vi "Send Get Temperature WAV.vi"(7 "Message Priority (Normal)":T1=enum."Normal", 8 "error in":errorcluster, 10 "Source":string, 11 "Message Enqueuer":refnum<class "Message Enqueuer.lvclass">) -> (0 "error out":errorcluster, 1 "timed out?":bool, 2 "Reply":variant, 3 "Message Enqueuer out":refnum<class "Message Enqueuer.lvclass">)   [LabVIEW 2024, in "Thermometer Multichannel Worker.lvlib" / "Get Temperature WAV Msg.lvclass"]
doc: "This VI sends the message to an actor."
uses:
  Get Temperature WAV Msg.lvclass
  Get Temperature WAV Msg.lvclass/Get Temperature WAV Msg.ctl
  <vilib>/ActorFramework/Reply Msg/Reply Msg.lvclass
  C:/Program Files/National Instruments/LabVIEW 2025/vi.lib/ActorFramework/Reply Msg/Reply Msg.lvclass
  C:/Program Files/National Instruments/LabVIEW 2025/vi.lib/ActorFramework/Message/Message.lvclass
  D:/git/HAL/Source/Thermometer Multichannel Worker/Thermometer Multichannel Worker Messages/Get Temperature WAV Msg/Get Temperature WAV Msg.lvclass
  <vilib>/ActorFramework/Message Enqueuer/Message Enqueuer.lvclass
  <vilib>/ActorFramework/Message Enqueuer/Message Priority.ctl
panel:
  in  "timeout in ms (-1)":i32=-1
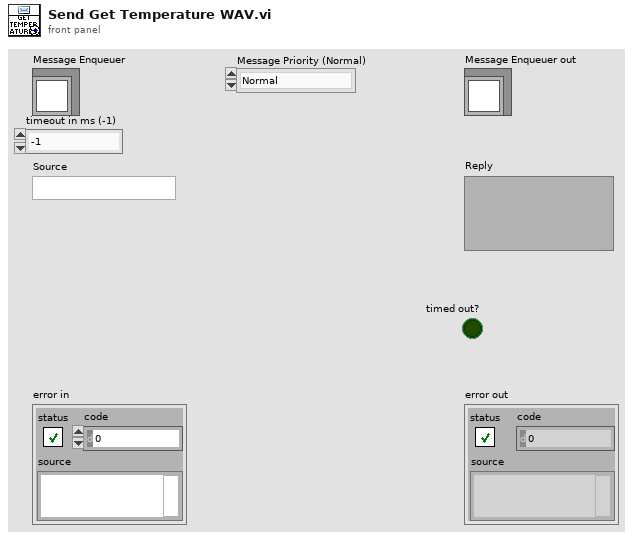
[diagram p1: front panel]
types:
  T1 = typedef "Actor Framework.lvlib/Message Enqueuer.lvclass/Message Priority.ctl" = enum16{"Low", "Normal", "High"}
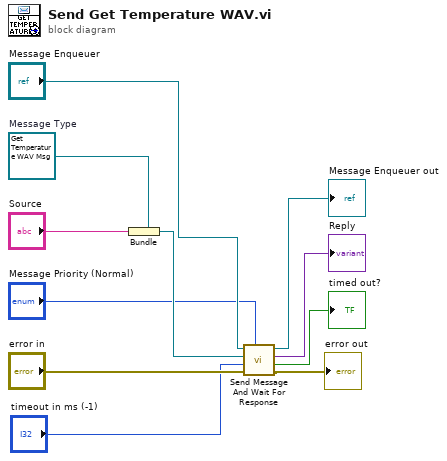
[diagram p0: block diagram]
diagram:
  w11 = refnum<class "Get Temperature WAV Msg.lvclass"> refnum  # Message Type
  n1 = Bundle(cluster=w11, "Source") -> (w7:refnum<class "Get Temperature WAV Msg.lvclass">)
  n2 = call <vilib>:"Send Message And Wait For Response.vi"("Message Priority (Normal)"="Message Priority (Normal)", "error in (no error)"="error in", "timeout in ms (-1)"="timeout in ms (-1)", "Original Message"=w7, "Message Enqueuer in"="Message Enqueuer") -> ("error out"=→"error out":errorcluster, "timed out?"=→"timed out?":bool, "Reply"=→"Reply":variant, "Message Enqueuer out"=→"Message Enqueuer out":refnum<class "Message Enqueuer.lvclass">)  [unwired: 3 in]
